vi "Set FFT - Spectral Parameters.vi"(0 "reference in":refnum<class "GSwFormDSP.lvclass">, 5 "error in (no error)":errorcluster, 7 "Spectral Function Parameters - User":T2 {"Window" items=["Rectangle"=0, "Hanning"=1, "Hamming"=2, "Blackman-Harris"=3, "Exact Blackman"=4, "Blackman"=5, "Flat Top"=6, "4 Term B-Harris "=7, "7 Term B-Harris"=8, "Low Sidelobe"=9, "Blackman Nuttall"=11, "Triangle"=30, "Bartlett-Hanning"=31, "Bohman"=32, "Parzen"=33, "Welch"=34, "Kaiser"=60, "Dolph-Chebyshev"=61, "Gaussian"=62]}) -> (14 "reference out":refnum<class "GSwFormDSP.lvclass">, 19 "error out":errorcluster)   [LabVIEW 2022 SP3, in "GSwFormDSP.lvclass"]
uses:
  GSwFormDSP.lvclass
  <vilib>/Analysis/4window.llb/windowTd.ctl
  <vilib>/Analysis/NI_AALPro.lvlib
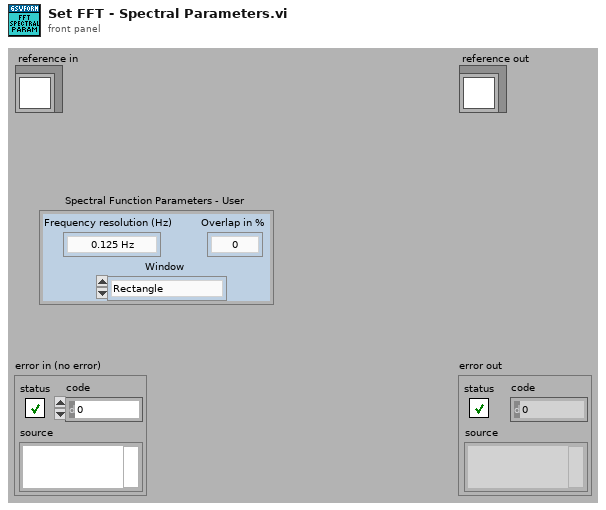
[diagram p1: front panel]
types:
  T1 = typedef "NI_AALPro.lvlib/windowTd.ctl" = u32
  T2 = cluster{"Frequency resolution (Hz)":enum16{"0.125 Hz", "0.25 Hz", "0.5 Hz", "1.0 Hz", "2.0 Hz", "4.0 Hz", "8.0 Hz", "16 Hz", "32 Hz", "64 Hz", "128 Hz"}, "Overlap in %":enum16{"0", "10", "20", "30", "40", "50", "60", "70", "80", "90"}, "Window":T1}
  T3 = typedef "GSwFormDSP.lvclass/ObjectAttributesRef.ctl" = refnum<data-value>
  T4 = typedef "GSwFormDSP.lvclass/ObjectAttributes.ctl" = cluster{"Wform Ref":refnum<data-value>, "Nb Signals":i32, "Spectral Function Parameters":T5, "FFT":waveform(cdb)[], "Nb FFT":i32, "Nb Averages":i32[], "Reference Indexes":i32[], "Response Indexes":i32[], "Coherence":waveform(dbl)[], "TDF Parameters":T6, "DAQ":cluster{"Duration (sec)":dbl, "Buffer Size (Samples)":i32, "Offset (Samples)":i32}, "Filter Impulse Response (TDF)":waveform(dbl), "Sound Playback":T7}
  T5 = typedef "GSwFormDSP.lvclass/Spectral Parameters.ctl" = cluster{"Frequency resolution (Hz)":dbl, "Overlap":dbl, "Window":T1}
  T6 = typedef "GSwFormDSP.lvclass/TDF Parameters.ctl" = cluster{"Filter":enum32{"Lowpass", "Highpass", "Bandpass", "Bandstop"}, "Type:":enum16{"Butterworth", "Chebyshev", "Inv Chebyshev", "Elliptic", "Bessel"}, "LP cutoff freq":dbl, "HP cutoff freq":dbl, "Order":i32, "passband ripple (dB)":dbl, "stopband attenuation (dB)":dbl, "Phaseless Filter":bool, "Include Fade IN and OUT":bool}
  T7 = typedef "GSwFormDSP.lvclass/Sound Playback.ctl" = cluster{"Timer start (ms)":u32, "task ID":T8, "Cursor Init Location (s)":dbl, "SC Volume":dbl}
  T8 = typedef "Sound Output Task ID.ctl" = u32
  T9 = enum16{"0.125 Hz", "0.25 Hz", "0.5 Hz", "1.0 Hz", "2.0 Hz", "4.0 Hz", "8.0 Hz", "16 Hz", "32 Hz", "64 Hz", "128 Hz"}
  T10 = enum16{"0", "10", "20", "30", "40", "50", "60", "70", "80", "90"}
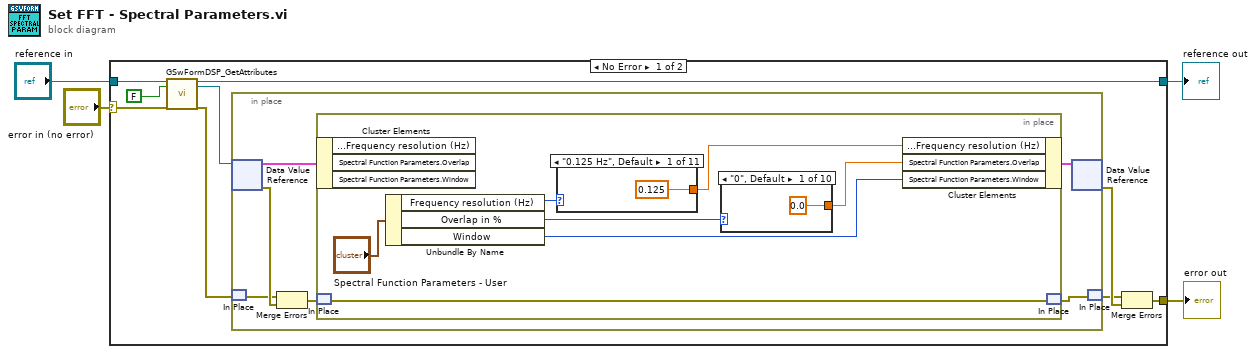
[diagram p0: block diagram]
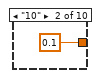
[diagram p2: hidden frame]
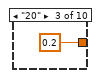
[diagram p3: hidden frame]
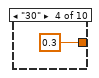
[diagram p4: hidden frame]
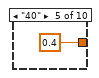
[diagram p5: hidden frame]
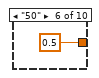
[diagram p6: hidden frame]
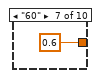
[diagram p7: hidden frame]
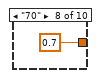
[diagram p8: hidden frame]
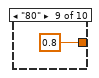
[diagram p9: hidden frame]
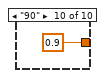
[diagram p10: hidden frame]
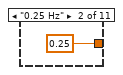
[diagram p11: hidden frame]
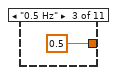
[diagram p12: hidden frame]
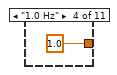
[diagram p13: hidden frame]
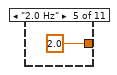
[diagram p14: hidden frame]
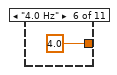
[diagram p15: hidden frame]
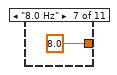
[diagram p16: hidden frame]
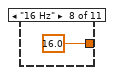
[diagram p17: hidden frame]
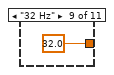
[diagram p18: hidden frame]
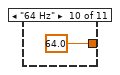
[diagram p19: hidden frame]
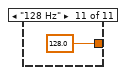
[diagram p20: hidden frame]
diagram:
  n1 = case shown="No Error" "error in (no error)" {
    selector: "error in (no error)" -> [w9 w49]
    tunnel: [w13 w49] -> w3
    tunnel: [w8 w48] -> w1
    tunnel: "reference in" -> [w11 w48]
    frame No Error {
      n2 = call "GSwFormDSP_GetAttributes.vi"("reference in"=w11, "return data? (T)"=FALSE, "error in (no error)"=w9) -> ("reference out"=w8:refnum<class "GSwFormDSP.lvclass">, "attributes ref"=w7:T3, "error out"=w6:errorcluster)  [unwired: 13 in, 1 out]
      n3 = in-place {
        n4 = in-place-dvr #1(w7) -> (w18:T4, w17:errorcluster)
        n5 = in-place-match #2(w6) -> (w16:errorcluster)
        n6 = Merge Errors(w16, w17) -> (w15:errorcluster)
        n7 = in-place {
          n8 = in-place-cluster #3(w18) -> ()  [unwired: 3 out]
          n9 = in-place-match #4(w15) -> (w20:errorcluster)
          n10 = Unbundle By Name("Spectral Function Parameters - User") -> ("Frequency resolution (Hz)"=w25:T9, "Overlap in %"=w23:T10, "Window"=w21:T1)
          n11 = case shown="\"0.125 Hz\", Default" w25 {
            tunnel: [0.125 ("Spectral Function Parameters.Frequency resolution (Hz)") 0.25 ("Spectral Function Parameters.Frequency resolution (Hz)") 0.5 ("Spectral Function Parameters.Frequency resolution (Hz)") 1.0 ("Spectral Function Parameters.Frequency resolution (Hz)") 2.0 ("Spectral Function Parameters.Frequency resolution (Hz)") 4.0 ("Spectral Function Parameters.Frequency resolution (Hz)") 8.0 ("Spectral Function Parameters.Frequency resolution (Hz)") 16.0 ("Spectral Function Parameters.Frequency resolution (Hz)") 32.0 ("Spectral Function Parameters.Frequency resolution (Hz)") 64.0 ("Spectral Function Parameters.Frequency resolution (Hz)") 128.0 ("Spectral Function Parameters.Frequency resolution (Hz)")] -> w24
            frame "0.125 Hz", Default {
            }
            frame "0.25 Hz" {
            }
            frame "0.5 Hz" {
            }
            frame "1.0 Hz" {
            }
            frame "2.0 Hz" {
            }
            frame "4.0 Hz" {
            }
            frame "8.0 Hz" {
            }
            frame "16 Hz" {
            }
            frame "32 Hz" {
            }
            frame "64 Hz" {
            }
            frame "128 Hz" {
            }
          }
          n12 = case shown="\"0\", Default" w23 {
            tunnel: [0.0 ("Spectral Function Parameters.Frequency resolution (Hz)") 0.1 ("Spectral Function Parameters.Frequency resolution (Hz)") 0.2 ("Spectral Function Parameters.Frequency resolution (Hz)") 0.3 ("Spectral Function Parameters.Frequency resolution (Hz)") 0.4 ("Spectral Function Parameters.Frequency resolution (Hz)") 0.5 ("Spectral Function Parameters.Frequency resolution (Hz)") 0.6 ("Spectral Function Parameters.Frequency resolution (Hz)") 0.7 ("Spectral Function Parameters.Frequency resolution (Hz)") 0.8 ("Spectral Function Parameters.Frequency resolution (Hz)") 0.9 ("Spectral Function Parameters.Frequency resolution (Hz)")] -> w22
            frame "0", Default {
            }
            frame "10" {
            }
            frame "20" {
            }
            frame "30" {
            }
            frame "40" {
            }
            frame "50" {
            }
            frame "60" {
            }
            frame "70" {
            }
            frame "80" {
            }
            frame "90" {
            }
          }
          n13 = in-place-cluster #3("Spectral Function Parameters.Frequency resolution (Hz)"=w24, "Spectral Function Parameters.Overlap"=w22, "Spectral Function Parameters.Window"=w21) -> (w19:T4)
          n14 = in-place-match #4(w20) -> (w14:errorcluster)
        }
        n15 = in-place-dvr #1(w19) -> (w12:errorcluster)  [unwired: 1 out]
        n16 = in-place-match #2(w14) -> (w5:errorcluster)
      }
      n17 = Merge Errors(w5, w12) -> (w13:errorcluster)
    }
    frame Error {
    }
  }
  "error out" <- w3
  "reference out" <- w1
